vi "dfd_C Check File Existence.vi"(6 "confirm?":bool=TRUE, 8 "error in (no error)":errorcluster, 9 "filter name":string, 10 "dest path":path) -> (0 "error out":errorcluster, 1 "filter name out":string, 2 "dest file refs":T1)   [LabVIEW 2017, in "NI_DigFilterLicensed.lvlib"]
uses:
  <vilib>/addons/Digital Filter Design/NI_DigFilterLicensed.lvlib
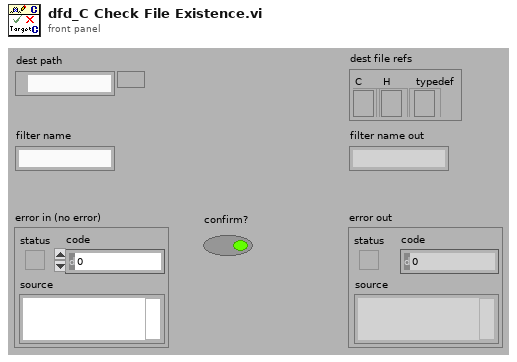
[diagram p1: front panel]
types:
  T1 = cluster{"C":refnum<file>, "H":refnum<file>, "typedef":refnum<file>}
  T2 = enum16{"open", "replace", "create", "open or create", "replace or create", "replace or create with confirmation"}
  T3 = cluster{"refnum out":refnum<file>, "refnum out":refnum<file>, "refnum out":refnum<file>}
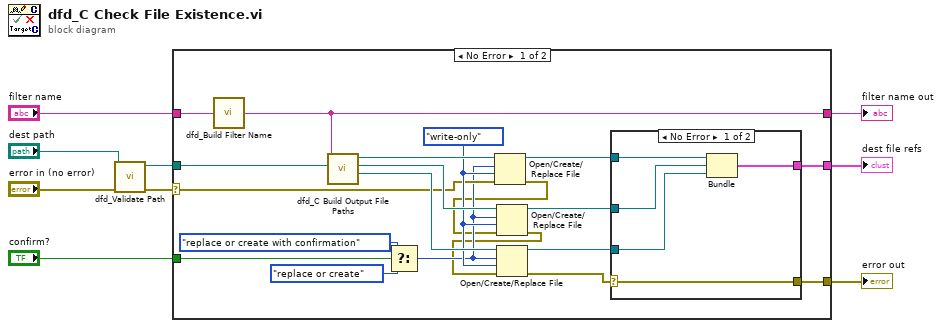
[diagram p0: block diagram]
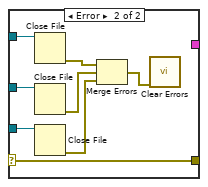
[diagram p2: hidden frame]
diagram:
  n1 = call <vilib>:"dfd_Validate Path.vi"("error in (no error)"="error in (no error)", "path in"="dest path") -> ("error out"=w4:errorcluster, "path out"=w6:path)  [unwired: 8 out]
  n2 = case shown="No Error" w4 {
    selector: w4 -> [w19 w43]
    tunnel: "filter name" -> [w29 _]
    tunnel: w6 -> [w28 _]
    tunnel: [w27 _] -> w5
    tunnel: "confirm?" -> [w25 _]
    tunnel: [w14 _] -> w1
    tunnel: [w13 w43] -> w2
    frame No Error {
      w20 = enum16{"read/write", "read-only", "write-only"}."write-only" ("access (0:read/write)")
      n3 = call <vilib>:"dfd_Build Filter Name.vi"("filter name in"=w29) -> ("filter name out"=w27:string)
      n4 = call <vilib>:"dfd_C Build Output File Paths.vi"("destination folder"=w28, "filter name"=w27) -> ("typedef path"=w21:path, "H path"=w22:path, "C path"=w23:path)  [unwired: 7 out]
      n5 = Select(t=T2."replace or create with confirmation" ("operation (0:open)"), s=w25, f=T2."replace or create" ("operation (0:open)")) -> (s? t:f=w18:T2)
      n6 = Open/Create/Replace File(file path (use dialog)=w23, error in=w19, operation (0:open)=w18, access (0:read/write)=w20) -> (refnum out=w17:refnum<file>, error out=w12:errorcluster)  [unwired: 3 out]
      n7 = Open/Create/Replace File(file path (use dialog)=w22, error in=w12, operation (0:open)=w18, access (0:read/write)=w20) -> (refnum out=w16:refnum<file>, error out=w11:errorcluster)  [unwired: 3 out]
      n8 = Open/Create/Replace File(file path (use dialog)=w21, error in=w11, operation (0:open)=w18, access (0:read/write)=w20) -> (refnum out=w15:refnum<file>, error out=w10:errorcluster)  [unwired: 3 out]
      n9 = case shown="No Error" w10 {
        selector: w10 -> [w34 w35]
        tunnel: w17 -> [w33 w42]
        tunnel: w16 -> [w32 w41]
        tunnel: w15 -> [w31 w40]
        tunnel: [w34 w35] -> w13
        tunnel: [w30 _] -> w14
        frame No Error {
          n10 = Bundle("refnum out"=w33, "refnum out"=w32, "refnum out"=w31) -> (w30:T3)  [unwired: 1 out]
        }
        frame Error {
          n11 = Close File(refnum=w42) -> (error out=w37:errorcluster)  [unwired: 1 in, 1 out]
          n12 = Close File(refnum=w41) -> (error out=w38:errorcluster)  [unwired: 1 in, 1 out]
          n13 = Close File(refnum=w40) -> (error out=w39:errorcluster)  [unwired: 1 in, 1 out]
          n14 = Merge Errors(w37, w38, w39) -> (w36:errorcluster)
          n15 = call <vilib>:"Clear Errors.vi"("error in (no error)"=w36) -> ()  [unwired: 1 in, 6 out]
        }
      }
    }
    frame Error {
    }
  }
  "error out" <- w2
  "filter name out" <- w5
  "dest file refs" <- w1
